vi "Launch Async Process.vi"(8 "error in (no error)":errorcluster, 11 "MQTT_Base in":refnum<class "MQTT_Base.lvclass">) -> ()   [LabVIEW 2013, in "MQTT Base.lvlib" / "MQTT_Base.lvclass"]
uses:
  MQTT_Base.lvclass
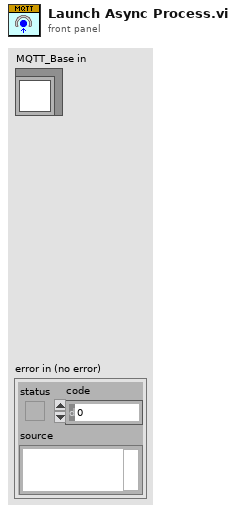
[diagram p1: front panel]
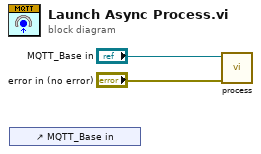
[diagram p0: block diagram]
diagram:
  n1 = control-ref of="MQTT_Base in"() -> ()  [unwired: 1 out]
  n2 = call-dynamic "process.vi"("error in (no error)"="error in (no error)", "MQTT_Base in"="MQTT_Base in") -> ()  [unwired: 9 in, 1 out]
